vi "checkFinishNormalDefensiveWithDuelistPlay.vi"(8 "error in (no error)":errorcluster, 10 "Game":refnum<class "Game.lvclass">, 11 "NormalDefensiveWithDuelistPlay in":refnum<class "NormalDefensiveWithDuelistPlay.lvclass">) -> (0 "error out":errorcluster, 2 "Boolean":bool, 3 "NormalDefensiveWithDuelistPlay out":refnum<class "NormalDefensiveWithDuelistPlay.lvclass">)   [LabVIEW 2018, in "NormalDefensiveWithDuelistPlay.lvclass"]
uses:
  NormalDefensiveWithDuelistPlay.lvclass
  Game_class/Game.lvclass
  Referee_class/command_interpreted.ctl
  Game_class/Game.lvclass/Game.ctl
  Events_class/Events.lvclass/Events.ctl
  Object_class/Object.lvclass/Object.ctl
  Ball_class/Ball.lvclass/Ball.ctl
  Referee_class/Referee.lvclass/Referee.ctl
  Game_class/Read Referee.vi
  Game_class/Read EventsRef.vi
  Events_class/Read ball_out.vi
  Referee_class/Read command_interpreted.vi
  Game_class/Read BallRef.vi
  Game_class/Read Parameters.lvclass.vi
  Game_class/Read FieldRef.vi
  Object_class/Read x.vi
  Object_class/Read y.vi
  Ball_class/Read v_x.vi
  Ball_class/Read v_y.vi
  Events_class/Read ball_inside_our_goalie_area.vi
  Ball_class/Ball.lvclass
  C:/Users/anton/Desktop/roboime/dar push/SSL_AI/SSL_AI/Object_class/Object.lvclass
  Events_class/Events.lvclass
  Parameters_class/Parameters.lvclass
  Field_class/Field.lvclass
  Referee_class/Referee.lvclass
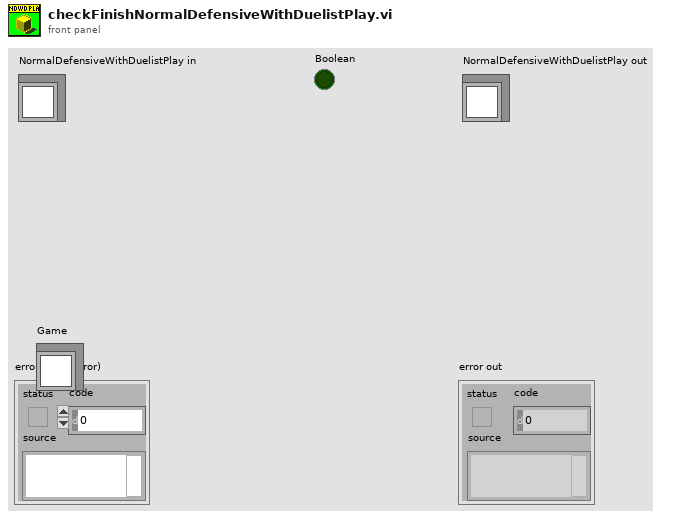
[diagram p1: front panel]
types:
  T1 = typedef "command_interpreted.ctl" = enum16{"Goal Ally", "Goal Enemy", "Ball Placement Enemy", "Ball Placement Ally", "Normal Half Time", "Extra Time  Break", "Extra Half Time", "None", "Post Game", "PKA Normal Start", "Prepare Kickoff Ally", "PKE Normal Start", "Prepare Kickoff Enemy", "Force Start", "Halt", "Timeout", "Prepare Penalty Ally", "Prepare Penalty Enemy", "PPA NormalStart", "PPE Normal Start", "Indirect Free Ally", "Direct Free Enemy", "Direct Free Ally", "Indirect Free Enemy", "Stop"}
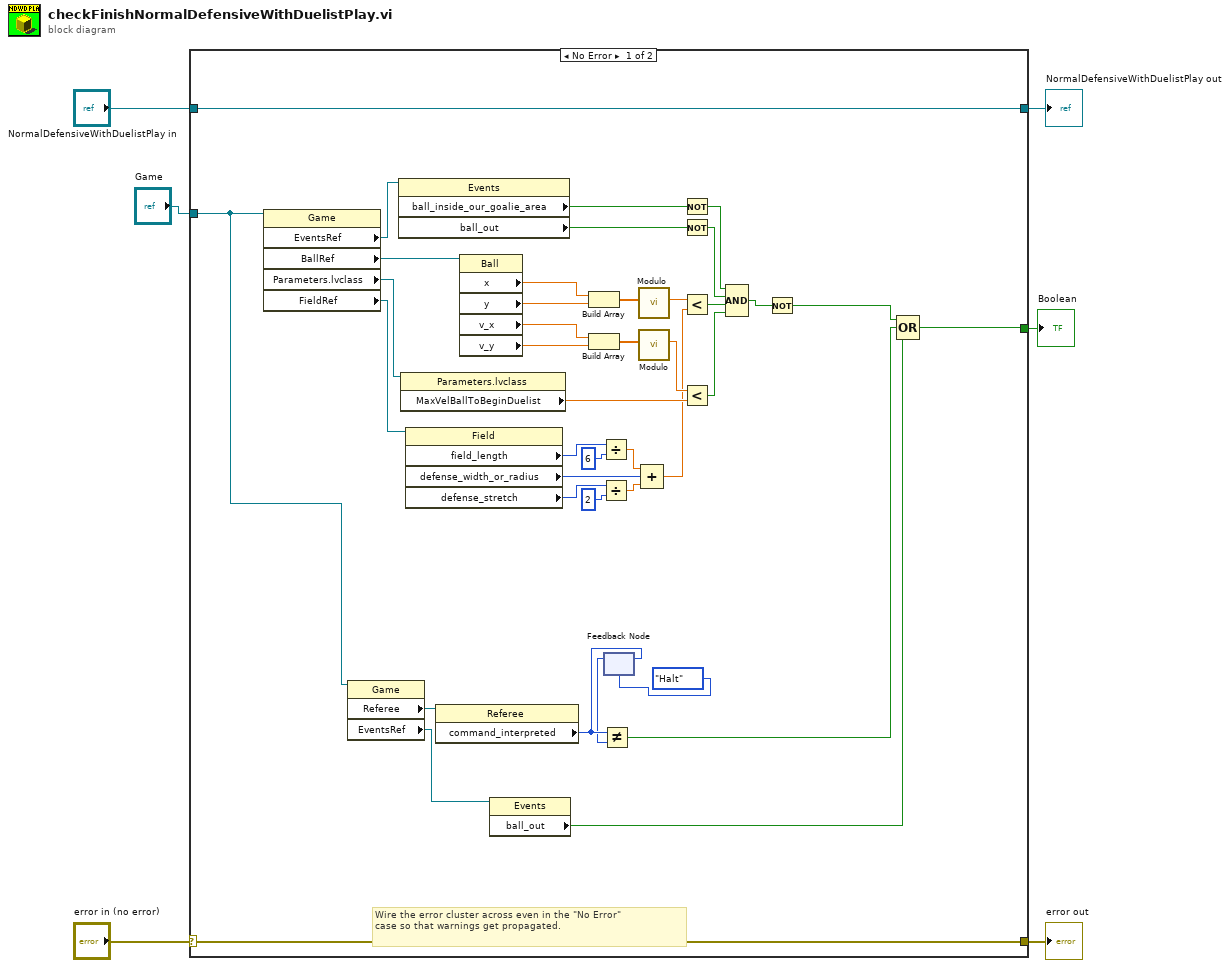
[diagram p0: block diagram]
diagram:
  n1 = case shown="No Error" "error in (no error)" {
    selector: "error in (no error)" -> [w45 w48]
    tunnel: [w45 w48] -> w5
    tunnel: [w46 w47] -> w3
    tunnel: "NormalDefensiveWithDuelistPlay in" -> [w46 w47]
    tunnel: "Game" -> [w12 _]
    tunnel: [w8 _] -> w1
    frame No Error {
      # "Wire the error cluster across even in the \"No Error\"\ncase so that warnings get propagated."
      n2 = property class="Game"(reference=w12) -> ("EventsRef"=w44:refnum<class "Events.lvclass">, "BallRef"=w39:refnum<class "Ball.lvclass">, "Parameters.lvclass"=w35:refnum<class "Parameters.lvclass">, "FieldRef"=w29:refnum<class "Field.lvclass">)  [unwired: 1 in, 2 out]
      n3 = property class="Game"(reference=w12) -> ("Referee"=w15:refnum<class "Referee.lvclass">, "EventsRef"=w10:refnum<class "Events.lvclass">)  [unwired: 1 in, 2 out]
      n4 = property class="Events"(reference=w44) -> ("ball_inside_our_goalie_area"=w43:bool, "ball_out"=w42:bool)  [unwired: 1 in, 2 out]
      n5 = property class="Parameters.lvclass"(reference=w35) -> ("MaxVelBallToBeginDuelist"=w30:dbl)  [unwired: 1 in, 2 out]
      n6 = property class="Field"(reference=w29) -> ("field_length"=w28:i32, "defense_width_or_radius"=w25:i32, "defense_stretch"=w23:i32)  [unwired: 1 in, 2 out]
      n7 = property class="Referee"(reference=w15) -> ("command_interpreted"=w14:T1)  [unwired: 1 in, 2 out]
      n8 = property class="Ball"(reference=w39) -> ("x"=w38:dbl, "y"=w37:dbl, "v_x"=w34:dbl, "v_y"=w33:dbl)  [unwired: 1 in, 2 out]
      n9 = property class="Events"(reference=w10) -> ("ball_out"=w9:bool)  [unwired: 1 in, 2 out]
      n10 = Build Array(w38, w37) -> (w36:dbl[])
      n11 = Build Array(w34, w33) -> (w32:dbl[])
      n12 = Divide(x=w28, y=6) -> (x/y=w26:dbl)
      n13 = Divide(x=w23, y=2) -> (x/y=w22:dbl)
      n14 = feedback #1(command_interpreted."Halt" ("command_interpreted")) -> (w7:T1)
      n15 = Not Equal?(x=w14, y=w7) -> (x != y?=w11:bool)
      n16 = feedback-in #1(w14) -> ()
      n17 = call "Modulo.vi"("2D vector"=w36) -> ("Modulo"=w21:dbl)  [unwired: 10 in]
      n18 = call "Modulo.vi"("2D vector"=w32) -> ("Modulo"=w31:dbl)  [unwired: 10 in]
      n19 = Compound Arithmetic op=ADD(w26, w25, w22) -> (w20:dbl)
      n20 = Not(x=w43) -> (.not. x?=w41:bool)
      n21 = Not(x=w42) -> (.not. x?=w40:bool)
      n22 = Less?(x=w21, y=w20) -> (x < y?=w19:bool)
      n23 = Less?(x=w31, y=w30) -> (x < y?=w18:bool)
      n24 = Compound Arithmetic op=AND(w41, w40, w19, w18) -> (w17:bool)
      n25 = Not(x=w17) -> (.not. x?=w16:bool)
      n26 = Compound Arithmetic op=OR(w16, w11, w9) -> (w8:bool)
    }
    frame Error {
    }
  }
  "error out" <- w5
  "NormalDefensiveWithDuelistPlay out" <- w3
  "Boolean" <- w1
